vi "Package Data.vi"(8 "error in":errorcluster, 10 "DataIn":string, 11 "Alicat Data in":refnum<class "Alicat Data.lvclass">) -> (0 "error out":errorcluster, 3 "Alicat Data out":refnum<class "Alicat Data.lvclass">)   [LabVIEW 2014, in "Alicat Lib.lvlib" / "Alicat Data.lvclass"]
uses:
  Alicat Data.lvclass
  Alicat Data.lvclass/Alicat Data.ctl
  Read Type.vi
  reusable/Data/Data.lvlibp/Write measTime.vi
  reusable/General/Atmospheric/Atmospheric Constants.vi
  reusable/General/Atmospheric/Atmospheric Library.lvlib
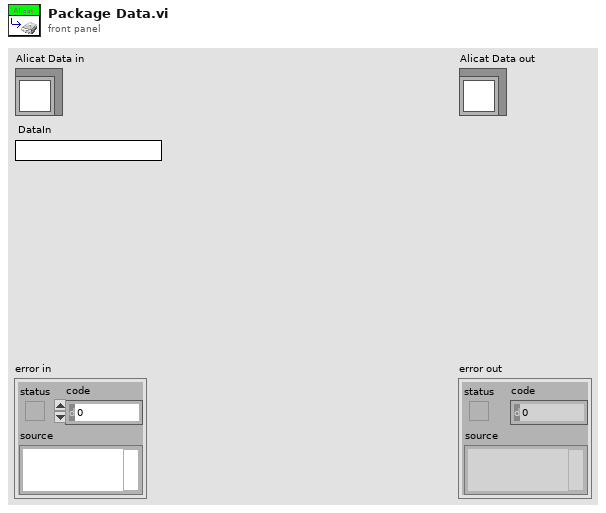
[diagram p1: front panel]
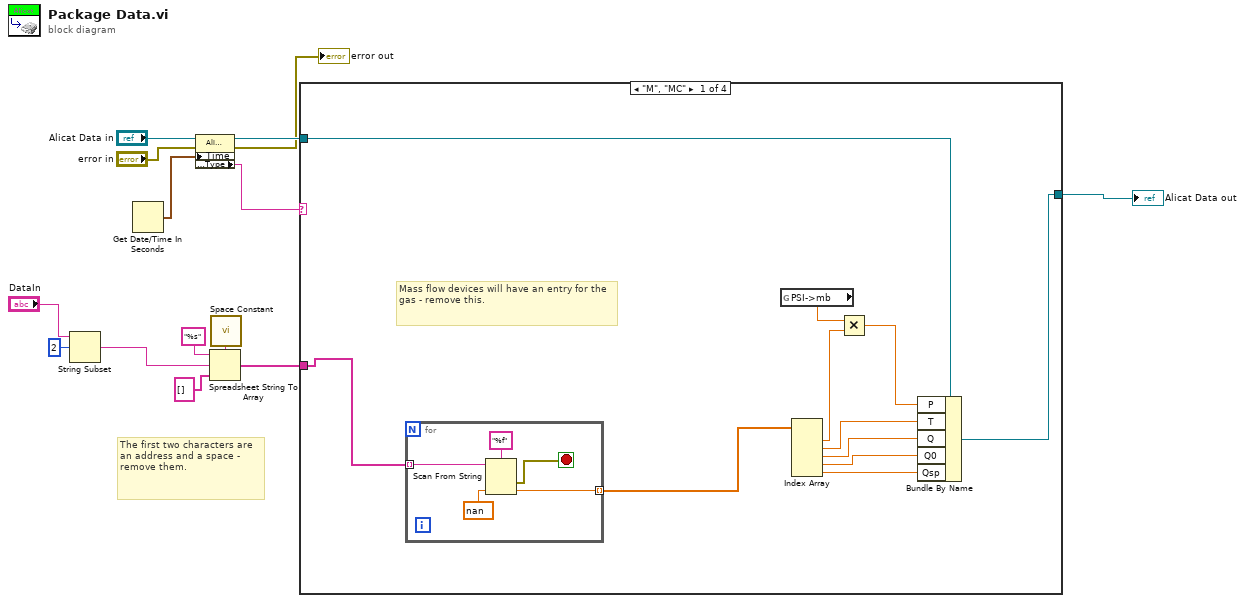
[diagram p0: block diagram]
diagram:
  # "The first two characters are an address and a space - remove them."
  n1 = String Subset(string="DataIn", offset (0)=2) -> (substring=w2:string)  [unwired: 1 in]
  n2 = Get Date/Time In Seconds() -> (seconds since 1Jan1904=w13:timestamp)
  n3 = property class="Alicat Data"(reference="Alicat Data in", error in="error in", "Time"=w13) -> (reference out=w10:refnum<class "Alicat Data.lvclass">, error out=→"error out":errorcluster, "Accessors:Type"=w11:string)
  n4 = call <vilib>:"Space Constant.vi"() -> ("String"=w6:string)
  n5 = Spreadsheet String To Array(delimiter (Tab)=w6, format string="%s", spreadsheet string=w2, array type (2D Dbl)=string[] []) -> (array=w5:string[])
  n6 = case shown="\"M\", \"MC\"" w11 {
    tunnel: w10 -> [w19 w31 w32 w33]
    tunnel: [w18 w31 w32 w33] -> w9
    tunnel: w5 -> [w17 _ _ _]
    frame "M", "MC" {
      # "Mass flow devices will have an entry for the gas - remove this."
      n7 = for {
        tunnel: w17 -> [w28] mode=indexing
        tunnel: [w26] -> w16 mode=indexing
        stop <- w27 stop-if-true
        n8 = Scan From String(format string="%f", input string=w28, default 1=sgl nan ("default value 1")) -> (error out=w27:errorcluster, output 1=w26:sgl)  [unwired: 2 in, 2 out]
      }
      n9 = global read "Atmospheric Constants.vi" "PSI->mb"() -> (w20:sgl)
      n10 = Index Array(array=w16) -> (element #1=w24:sgl, element #2=w23:sgl, element #3=w22:sgl, element #4=w21:sgl, element #5=w15:sgl)  [unwired: 5 in]
      n11 = Multiply(x=w20, y=w24) -> (x*y=w25:sgl)
      n12 = Bundle By Name(cluster=w19, "P"=w25, "T"=w23, "Q"=w22, "Q0"=w21, "Qsp"=w15) -> (w18:refnum<class "Alicat Data.lvclass">)
    }
    frame "VC" {
    }
    frame "V" {
    }
    frame "Null", Default {
    }
  }
  "Alicat Data out" <- w9
